vi "Configure Third Order Intercept (Measurement Setup).vi"(0 "VISA resource name":refnum<visa-resource-name>, 5 "Third Order Search (1:On)":i32(ring)=1 items=["Off", "On"], 7 "Low Tone (1:On)":i32(ring)=1 items=["Off", "On"], 9 "Frequency (1125000000Hz)":dbl=1125000000.0 min=-100000000.0 max=43100000000.0, 11 "error in (no error)":errorcluster) -> (4 "VISA resource name out":refnum<visa-resource-name>, 15 "error out":errorcluster)   [LabVIEW 2020, in "Anritsu Signal Analyzer Series.lvlib"]
doc: "Sets the TOI measurement parameters."
uses:
  Anritsu Signal Analyzer Series.lvlib
panel:
  # "Hz"
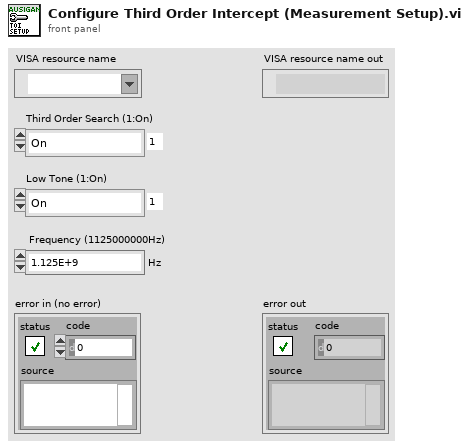
[diagram p1: front panel]
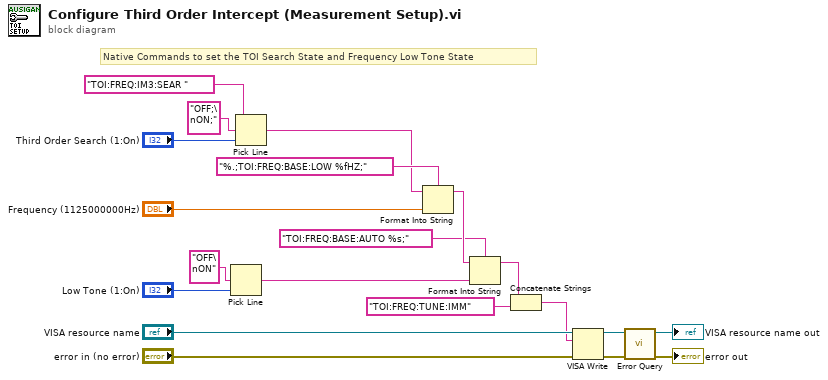
[diagram p0: block diagram]
diagram:
  # "Native Commands to set the TOI Search State and Frequency Low Tone State"
  n1 = Pick Line(multi-line string="OFF\nON" ("複数行文字列"), line index="Low Tone (1:On)") -> (output string=w1:string)  [unwired: 1 in]
  n2 = Pick Line(string ("")="TOI:FREQ:IM3:SEAR " ("_CommandSet"), multi-line string="OFF;\nON;" ("複数行文字列"), line index="Third Order Search (1:On)") -> (output string=w4:string)
  n3 = Format Into String(format string="%.;TOI:FREQ:BASE:LOW %fHZ;" ("Format String"), initial string=w4, "Frequency (1125000000Hz)") -> (resulting string=w12:string)  [unwired: 1 in, 1 out]
  n4 = Format Into String(format string="TOI:FREQ:BASE:AUTO %s;" ("_CommandSet"), initial string=w12, w1) -> (resulting string=w7:string)  [unwired: 1 in, 1 out]
  n5 = Concatenate Strings(w7, "TOI:FREQ:TUNE:IMM" ("_CommandSet")) -> (w6:string)
  n6 = VISA Write(VISA resource name="VISA resource name", write buffer=w6, error in (no error)="error in (no error)") -> (VISA resource name out=w10:refnum<visa-resource-name>, error out=w9:errorcluster)  [unwired: 1 out]
  n7 = call "Error Query.vi"("error in (no error)"=w9, "VISA resource name"=w10) -> ("error out"=→"error out":errorcluster, "VISA resource name out"=→"VISA resource name out":refnum<visa-resource-name>)  [unwired: 6 in, 2 out]
